vi "SETMIXTUREdll_Test.vi"(8 "error in (no error)":errorcluster) -> (0 "error out":errorcluster, 3 "Passed?":bool)   [LabVIEW 2021]
panel:
  out "ierr":i32=101
  out "z":dbl[](array[numeric])
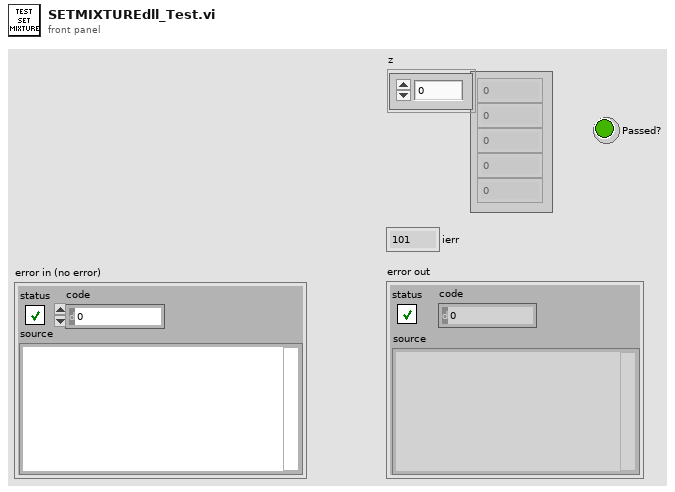
[diagram p1: front panel]
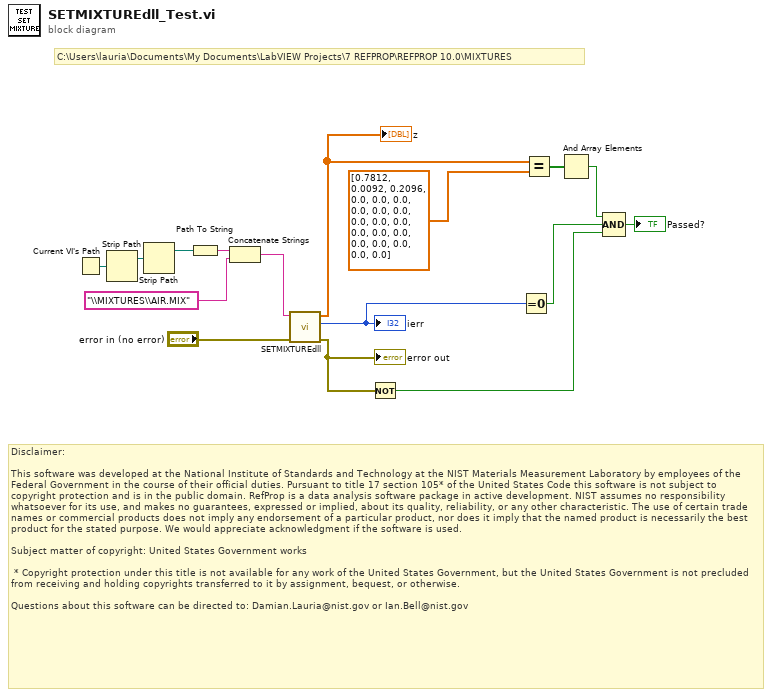
[diagram p0: block diagram]
diagram:
  # "C:\\Users\\lauria\\Documents\\My Documents\\LabVIEW Projects\\7 REFPROP\\REFPROP 10.0\\MIXTURES"
  # "Disclaimer:\n\nThis software was developed at the National Institute of Standards and Technology at the NIST Materials Measurement Laboratory by employees of the Federal Government in the course of their official duties. Pursuant to title 17 section 105* of the United States Code this software is not subject to copyright protection and is in the public domain. RefProp is a data analysis software package in active development. NIST assumes no responsibility whatsoever for its use, and makes no guarantees, expressed or implied, about its quality, reliability, or any other characteristic. The use of certain trade names or commercial products does not imply any endorsement of a particular product, nor does it imply that the named product is necessarily the best product for the stated purpose. We would appreciate acknowledgment if the software is used.\n \nSubject matter of copyright: United States Government works\n  \n * Copyright protection under this title is not available for any work of the United States Government, but the United States Government is not precluded from receiving and holding copyrights transferred to it by assignment, bequest, or otherwise.\n\nQuestions about this software can be directed to: Damian.Lauria@nist.gov or Ian.Bell@nist.gov"
  n1 = Current VI's Path() -> (path=w6:path)
  n2 = Strip Path(path=w6) -> (stripped path=w5:path)  [unwired: 1 out]
  n3 = Strip Path(path=w5) -> (stripped path=w4:path)  [unwired: 1 out]
  n4 = Path To String(path=w4) -> (string=w3:string)
  n5 = Concatenate Strings(w3, "\\MIXTURES\\AIR.MIX" ("string")) -> (w1:string)
  n6 = call "SETMIXTUREdll.vi"("error in (no error)"="error in (no error)", "hmixnme"=w1) -> ("error out"=w12:errorcluster, "ierr"=w15:i32, "z"=w14:dbl[])  [unwired: 7 in]
  "error out" <- w12
  "z" <- w14
  "ierr" <- w15
  n7 = Not(x=w12) -> (.not. x?=w11:bool)
  n8 = Equal To 0?(x=w15) -> (x = 0?=w10:bool)
  n9 = Equal?(x=w14, y=dbl[] [0.7812, 0.0092, 0.2096, 0.0, 0.0, 0.0, 0.0, 0.0, 0.0, 0.0, 0.0, 0.0, 0.0, 0.0, 0.0, 0.0, 0.0, 0.0, 0.0, 0.0] ("z")) -> (x = y?=w9:bool[])
  n10 = And Array Elements(Boolean array=w9) -> (logical AND=w8:bool)
  n11 = Compound Arithmetic op=AND(w8, w10, w11) -> (→"Passed?":bool)
